vi "myRIO_BRig_RT_dataCurrent_LorR.vi"() -> (2 "output_LorR":i32)   [LabVIEW 2014]
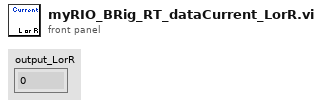
[diagram p1: front panel]
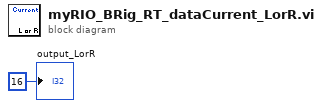
[diagram p0: block diagram]
diagram:
  "output_LorR" <- 16 ("output_iBlock")
